vi "CheckBoundsAndIncrement.vi"(10 "Increment":T1, 11 "Rectangle In":T1) -> (3 "Rectangle Out":T1)   [LabVIEW 2020, in "Ants.lvclass"]
doc: "This VI adds <b>Increment</b> to <b>Rectangle In</b>, checks that both axes have at least 1 corner in the range 1-31 (i.e. rectangle in valid range), and returns the resulting rectangle.\n\nIf the resulting rectangle is invalid, this VI returns <b>Rectangle Input</b> unmodified."
uses:
  Ants.lvclass
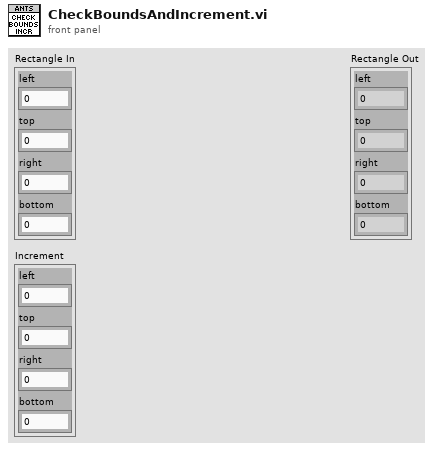
[diagram p1: front panel]
types:
  T1 = cluster{"left":i16, "top":i16, "right":i16, "bottom":i16}
  T2 = cluster{"left":bool, "top":bool, "right":bool, "bottom":bool}
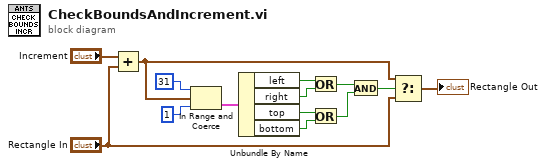
[diagram p0: block diagram]
diagram:
  n1 = Add(x="Increment", y="Rectangle In") -> (x+y=w1:T1)
  n2 = In Range and Coerce(upper limit=31, x=w1, lower limit=1) -> (In Range?=w12:T2)  [unwired: 1 out]
  n3 = Unbundle By Name(w12) -> ("left"=w11:bool, "right"=w10:bool, "top"=w9:bool, "bottom"=w8:bool)
  n4 = Or(x=w11, y=w10) -> (x .or. y?=w7:bool)
  n5 = Or(x=w9, y=w8) -> (x .or. y?=w6:bool)
  n6 = And(x=w7, y=w6) -> (x .and. y?=w5:bool)
  n7 = Select(t=w1, s=w5, f="Rectangle In") -> (s? t:f=→"Rectangle Out":T1)
